vi "Define_Last_Point_in_Subtrack-1.vi"(4 "[IN] Statuses":i16[](array[numeric])) -> (1 "[OUT] Index of Problem Point\nin Subtrack (Original)":i32)   [LabVIEW 2013]
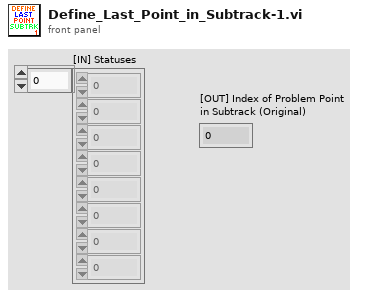
[diagram p1: front panel]
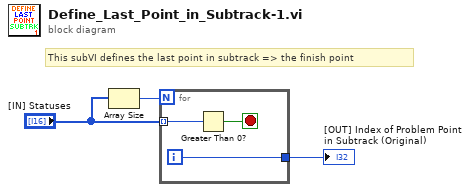
[diagram p0: block diagram]
diagram:
  # "This subVI defines the last point in subtrack => the finish point"
  n1 = Array Size(array="[IN] Statuses") -> (size(s)=w3:i32)
  n2 = for {
    N: w3 -> [_]
    tunnel: "[IN] Statuses" -> [w6] mode=indexing
    tunnel: [w4] -> w1
    i -> [w4]
    stop <- w5 stop-if-true
    n3 = Greater Than 0?(x=w6) -> (x > 0?=w5:bool)
  }
  "[OUT] Index of Problem Point\nin Subtrack (Original)" <- w1
